vi "Auto settings.vi"(8 "error in (no error)":errorcluster, 10 "PUT Settings":T1, 11 "Fixture in":refnum<class "Fixture.lvclass">) -> (0 "error out":errorcluster, 3 "Fixture out":refnum<class "Fixture.lvclass">)   [LabVIEW 2021, in "Fixture.lvclass"]
uses:
  Fixture.lvclass
  Fixture.lvclass/Fixture.ctl
  SubVIs/PUT_region.vi
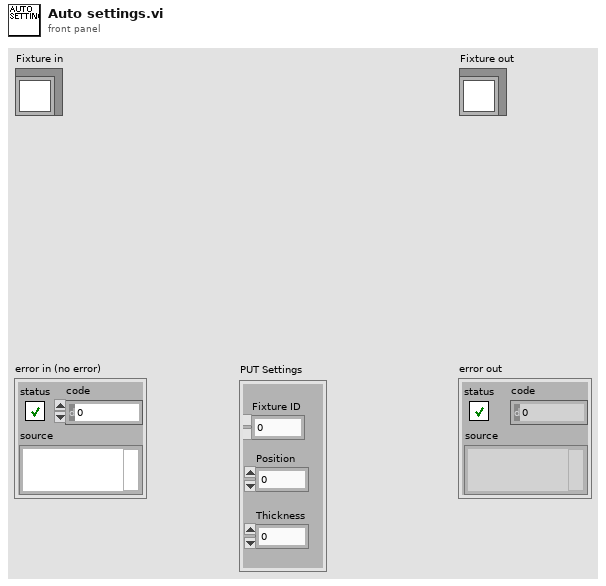
[diagram p1: front panel]
types:
  T1 = cluster{"Fixture ID":dbl, "Position":dbl, "Thickness":dbl}
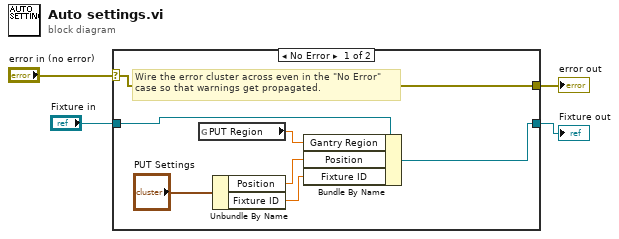
[diagram p0: block diagram]
diagram:
  n1 = case shown="No Error" "error in (no error)" {
    selector: "error in (no error)" -> [w11 w13]
    tunnel: [w11 w13] -> w3
    tunnel: [w9 w12] -> w1
    tunnel: "Fixture in" -> [w10 w12]
    frame No Error {
      # "Wire the error cluster across even in the \"No Error\"\ncase so that warnings get propagated."
      n2 = global read "PUT_region.vi" "PUT Region"() -> (w8:dbl)
      n3 = Unbundle By Name("PUT Settings") -> ("Position"=w6:dbl, "Fixture ID"=w5:dbl)
      n4 = Bundle By Name(cluster=w10, "Gantry Region"=w8, "Position"=w6, "Fixture ID"=w5) -> (w9:refnum<class "Fixture.lvclass">)
    }
    frame Error {
    }
  }
  "error out" <- w3
  "Fixture out" <- w1
